vi "tsflexray_set_frametrigger.vi"() -> ()   [LabVIEW 2014]
doc: "TSAPI(s32)tsflexray_set_frametrigger(const s32 AIdxChn,const ps32 AFrameLengthArray,const s32 AFrameNum,const PLIBTrigger_def AFrameTrigger,const s32 AFrameTriggerNum,const s32 ATimeoutMs);"
panel:
  out "路径输出":path
  in  "路径输入":path
  out "error out":errorcluster caption="错误输出"
  in  "error in (no error)":errorcluster caption="错误输入（无错误）"
  in  "ATimeoutMs":i32
  in  "AFrameTriggerNum":i32
  in  "AFrameTrigger":T1
  in  "AFrameNum":i32
  in  "AFrameLengthArray":i32
  in  "AIdxChn":i32
  out "function return":i32
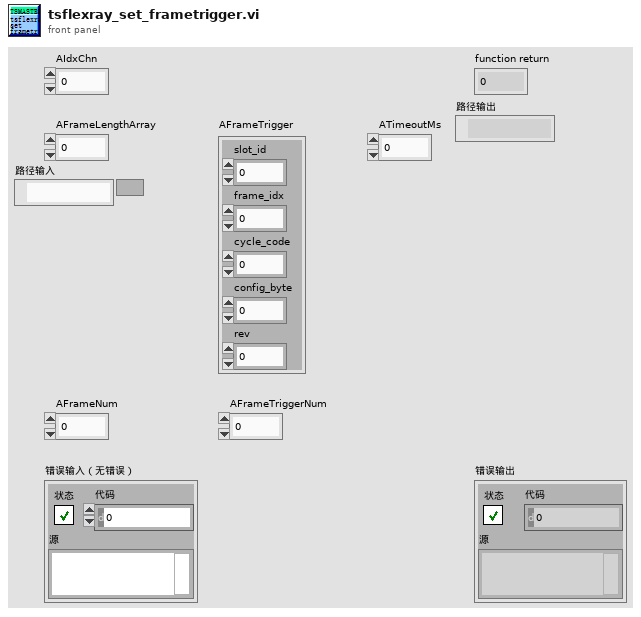
[diagram p1: front panel]
types:
  T1 = cluster{"slot_id":u32, "frame_idx":u8, "cycle_code":u8, "config_byte":u8, "rev":u8}
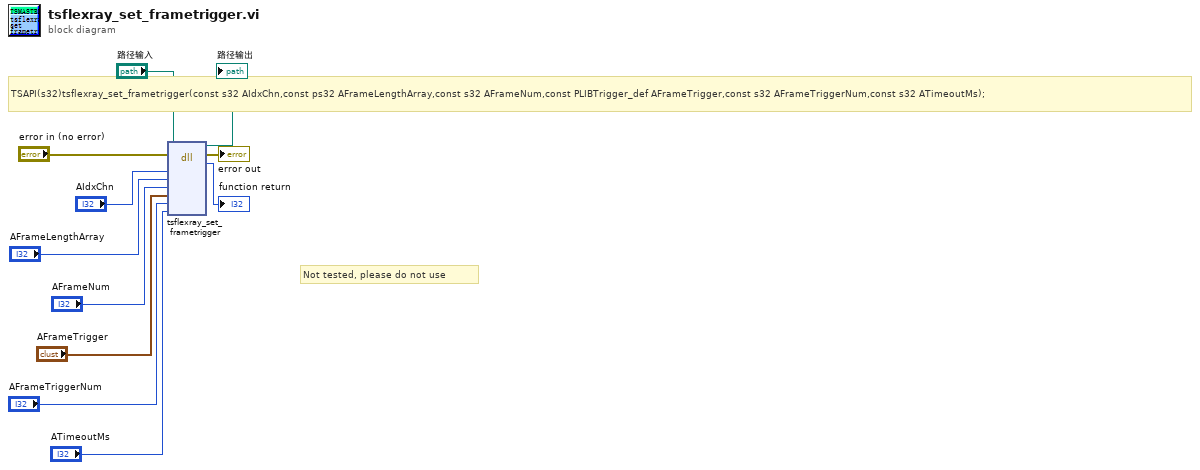
[diagram p0: block diagram]
diagram:
  # "Not tested, please do not use"
  # "TSAPI(s32)tsflexray_set_frametrigger(const s32 AIdxChn,const ps32 AFrameLengthArray,const s32 AFrameNum,const PLIBTrigger_def AFrameTrigger,const s32 AFrameTriggerNum,const s32 ATimeoutMs);"
  n1 = dll-call lib="D:/Work/LabVIEW Code/TSMaster Labview SDK/LabVIEW/LabVIEW-TSMasterAPI_CLN/TSMasterAPI_LabVIEW-2024-10-08 14-20-13/Not_organized_vi/TSMaster.*" fn="tsflexray_set_frametrigger"(path in="路径输入", error in="error in (no error)", "AIdxChn"="AIdxChn", "AFrameLengthArray"="AFrameLengthArray", "AFrameNum"="AFrameNum", "AFrameTrigger"="AFrameTrigger", "AFrameTriggerNum"="AFrameTriggerNum", "ATimeoutMs"="ATimeoutMs") -> (path out=→"路径输出":path, error out=→"error out":errorcluster, "返回类型"=→"function return":i32)  [unwired: 7 in]
